vi "motors_id.vi"() -> ()   [LabVIEW 2019]
uses:
  Control 1.ctl
  <vilib>/Analysis/Matrix/Datatypes/RealMatrix.ctl
  <vilib>/userDefined/High Color/IMAQdx.ctl
  <vilib>/Platform/TimedLoop/XDataNode/timing_clust.ctl
  <vilib>/Platform/TimedLoop/XDataNode/nitl_modes.ctl
  <vilib>/Platform/TimedLoop/XDataNode/wakeup.ctl
  <vilib>/myRIO/Instrument Drivers/Onboard IO/AO/typedefs/AO Reference.ctl
  <vilib>/myRIO/Common/Instrument Driver Framework/Utilities/typedefs/myRIO Generic Hardware Reference.ctl
  <vilib>/myRIO/Common/Instrument Driver Framework/Utilities/typedefs/Hardware Version Enum.ctl
  <vilib>/myRIO/Common/Instrument Driver Framework/Utilities/typedefs/myRIO v1.0 Reference.ctl
  <vilib>/myRIO/Common/Instrument Driver Framework/Utilities/typedefs/Generic FPGA Reference.ctl
  <vilib>/myRIO/Common/Instrument Driver Framework/myRIO v1.0/AO/typedefs/AO Channels List.ctl
  <vilib>/myRIO/Common/Instrument Driver Framework/myRIO v1.0/AO/typedefs/AO Channels Enum.ctl
  <vilib>/myRIO/Common/Instrument Driver Framework/Utilities/typedefs/Analog Scaling Constants List.ctl
  <vilib>/myRIO/Common/Instrument Driver Framework/Utilities/typedefs/Analog Scaling Constants.ctl
  <vilib>/userDefined/High Color/nirio_resource_hc.ctl
  <vilib>/myRIO/Common/Instrument Driver Framework/myRIO v1.0/Encoder/typedefs/Encoder Signal Mode.ctl
  <vilib>/myRIO/Instrument Drivers/Onboard IO/Encoder/typedefs/Encoder Reference.ctl
  <vilib>/myRIO/Common/Instrument Driver Framework/myRIO v1.0/Encoder/typedefs/Encoder Channels Enum.ctl
  <vilib>/myRIO/Common/Instrument Driver Framework/myRIO v1.0/Encoder/typedefs/Encoder Configuration v1.0.ctl
  <vilib>/myRIO/Common/Instrument Driver Framework/Utilities/vis/Is FPGA Ref Available.vi
  <vilib>/myRIO/Common/Instrument Driver Framework/myRIO v1.0/AO/vis/myRIO v1.1 Open AO.vi
  <vilib>/myRIO/Instrument Drivers/Onboard IO/AO/vis/Write.vi
  <vilib>/myRIO/Common/Instrument Driver Framework/myRIO v1.0/Encoder/vis/myRIO v1.1 Open Encoder.vi
  <vilib>/myRIO/Instrument Drivers/Onboard IO/Encoder/vis/Read.vi
  <vilib>/myRIO/Common/Instrument Driver Framework/Utilities/vis/Validate Channels.vi
  <vilib>/myRIO/Common/Instrument Driver Framework/myRIO v1.0/AO/vis/myRIO v1.0 Reserve AO.vi
  <vilib>/myRIO/Common/Instrument Driver Framework/myRIO v1.0/Encoder/vis/myRIO v1.0 Reserve Encoder.vi
  <vilib>/myRIO/Common/Instrument Driver Framework/myRIO v1.0/AO/vis/myRIO v1.0 Build MUX Configuration AO.vi
  <vilib>/myRIO/Common/Instrument Driver Framework/myRIO v1.0/Resource Manager/vis/myRIO v1.0 Reserve Channel List.vi
  <vilib>/myRIO/Common/Instrument Driver Framework/myRIO v1.0/Encoder/vis/myRIO v1.0 Build MUX Configuration Encoder.vi
  <vilib>/myRIO/Common/Instrument Driver Framework/myRIO v1.0/Resource Manager/vis/myRIO v1.0 Reserve Channel.vi
  <vilib>/myRIO/Common/Instrument Driver Framework/myRIO v1.0/Resource Manager/vis/myRIO v1.0 Unreserve Channel.vi
  <vilib>/myRIO/Common/Instrument Driver Framework/myRIO v1.0/Resource Manager/vis/myRIO v1.0 Create Configuration List.vi
  <vilib>/myRIO/Common/Instrument Driver Framework/myRIO v1.0/Resource Manager/vis/myRIO v1.0 Build Mutex Name.vi
  <vilib>/Utility/VariantDataType/GetNumericInfo.vi
  <vilib>/Utility/error.llb/Error Cluster From Error Code.vi
  <vilib>/myRIO/Common/Instrument Driver Framework/myRIO v1.0/myRIO v1.1 Open.vi
  <vilib>/myRIO/Common/Instrument Driver Framework/myRIO v1.0/AO/vis/myRIO v1.0 Get Scaling Constants AO.vi
  <vilib>/myRIO/Common/Instrument Driver Framework/Utilities/vis/IO Manager.vi
  <vilib>/myRIO/Common/Instrument Driver Framework/Utilities/vis/Configuration Manager.vi
  <vilib>/myRIO/Common/Instrument Driver Framework/myRIO v1.0/myRIO v1.0 Close.vi
  <vilib>/myRIO/Common/Instrument Driver Framework/myRIO v1.0/AO/vis/myRIO v1.0 Write AO.vi
  <vilib>/Utility/file.llb/Write Delimited Spreadsheet (DBL).vi
  <vilib>/myRIO/Common/Instrument Driver Framework/myRIO v1.0/Resource Manager/vis/myRIO v1.0 Configure IO.vi
  <vilib>/myRIO/Common/Instrument Driver Framework/myRIO v1.0/Encoder/vis/myRIO v1.0 Configure Encoder.vi
  <vilib>/myRIO/Common/Instrument Driver Framework/myRIO v1.0/Encoder/vis/myRIO v1.0 Read Encoder.vi
  <vilib>/platform/TimedLoop/XDataNode/XDataNode.xnode
  <vilib>/myRIO/Express VI/Onboard IO/AO/AO Express VI.xnode
  <vilib>/myRIO/Instrument Drivers/Onboard IO/AO/vis/myRIO AO Open.xnode
  <vilib>/myRIO/Express VI/Onboard IO/Encoder/Encoder Express VI.xnode
  <vilib>/myRIO/Instrument Drivers/Onboard IO/Encoder/vis/myRIO Encoder Open.xnode
  <vilib>/myRIO/Common/Instrument Driver Framework/myRIO v1.0/Encoder/typedefs/Encoder Count Direction Enum.ctl
  <vilib>/Platform/TimedLoop/XDataNode/XDNodeRunTimeDep.lvlib
  <vilib>/myRIO/Instrument Drivers/Onboard IO/AO/AO.lvlib
  <vilib>/vision/driver/NI_Vision_Acquisition_Software.lvlib
  <vilib>/myRIO/Instrument Drivers/Onboard IO/Encoder/Encoder.lvlib
  <vilib>/vision/NI_Vision_Development_Module.lvlib
  <vilib>/Analysis/Matrix/NI_Matrix.lvlib
panel:
  in  "x_a":dbl(slide) step=1.0 scale=-45.0..45.0
  in  "y_a":dbl(slide) step=1.0 scale=-45.0..45.0
  in  "record_name":string
  out "record":T1
  out "step_recorded":dbl
  in  "stop_recording":bool
  in  "start_recording":bool
  out "recording":bool
  out "record_t":dbl[](array[numeric])
  out "target_angle_y_a_target":dbl(knob) scale=-45.0..45.0
  out "target_angle_x_a_target":dbl(knob) scale=-45.0..45.0
  in  "p_ki":dbl=-1.0
  in  "p_kd":dbl=-2000.0
  in  "p_kp":dbl
  out "y_angle":dbl(knob) scale=-45.0..45.0
  out "x_angle":dbl(knob) scale=-45.0..45.0
  out "y_error":dbl
  out "x_error":dbl
  in  "y_target":dbl(slide) scale=-1.0..1.0
  in  "x_target":dbl(slide) scale=-1.0..1.0
  out "y":dbl
  out "x":dbl
  out "camera":T2(plugin-control)
  in  "threshold":cluster{"Lower value":sgl, "Upper value":sgl}={"Lower value"=189.0, "Upper value"=255.0} {"Upper value" format="%.2f"; "Lower value" format="%.2f"}
  out "threshold":T2(plugin-control)
  out "x-y":u32
  out "y_input":dbl
  in  "a_ki":dbl=0.0003
  out "y_angle_error":dbl
  in  "a_kd":T3=-2.0
  in  "a_kp":dbl=0.12
  out "x_angle_error":dbl
  in  "stop":bool
  out "x_input":dbl
  in  "reset":bool
  in  "dt":dbl=70.0
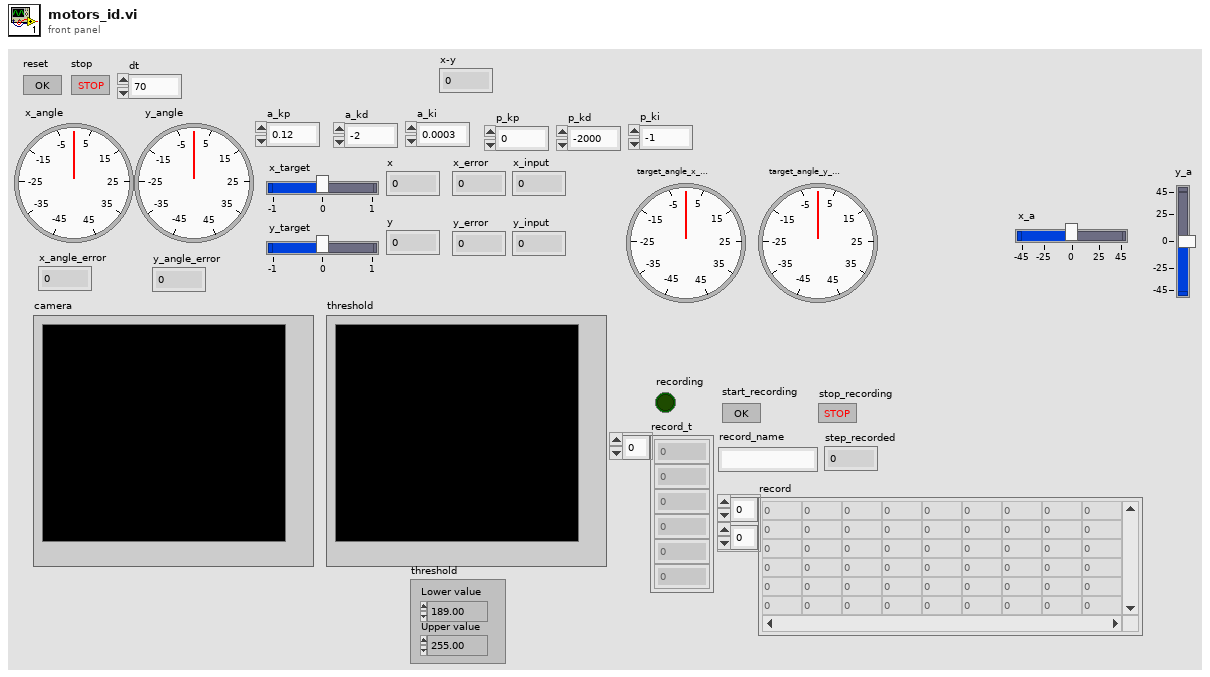
[diagram p1: front panel]
types:
  T1 = typedef "NI_Matrix.lvlib/RealMatrix.ctl" = dbl[][]
  T2 = typedef "IMAQ Image.ctl" = refnum<image>
  T3 = typedef "Control 1.ctl" = dbl
  T4 = typedef "IMAQdx.ctl" = refnum<k21>
  T5 = typedef "XDNodeRunTimeDep.lvlib/timing_clust.ctl" = cluster{"Expected End [f-1]":u64, "Actual End [f-1]":u64, "Finished Late? [f-1]":bool, "Expected End [i-1]":u64, "Actual End [i-1]":u64, "Finished Late? [i-1]":bool, "Expected Start [i]":u64, "Actual Start [i]":u64, "Expected Start [f]":u64, "Actual Start [f]":u64, "Source Name":string, "Structure Name":string, "Period":i64, "Deadline":i64, "Offset":i64, "Start":i64, "Priority":i32, "Timeout":i32, "Mode":T6, "Wakeup Reason":T7, "Error":errorcluster, "Source Type":string, "Secondary Source Type":string, "Global End Time":u64, "Global Start Time":u64, "Frame Duration":u64, "Iteration Duration":u64, "Assigned CPU":i32, "I/O Scan Engine Mode":u32}
  T6 = typedef "XDNodeRunTimeDep.lvlib/nitl_modes.ctl" = enum32{"No Change", "Process missed periods, maintain original phase", "Discard missed periods, maintain original phase", "Process missed periods, ignore original phase", "Discard missed periods, ignore original phase"}
  T7 = typedef "XDNodeRunTimeDep.lvlib/wakeup.ctl" = enum32{"Normal", "Aborted", "Asynchronous wakeup", "Timing source error", "Timed loop error", "Timeout"}
  T8 = typedef "Encoder.lvlib/Encoder Reference.ctl" = cluster{"myRIO Reference":T9, "Encoder Channels Enum":T13}
  T9 = typedef "myRIO Generic Hardware Reference.ctl" = cluster{"myRIO Model":T10, "myRIO Hardware Reference":T11}
  T10 = typedef "Hardware Version Enum.ctl" = enum16{"Unknown", "myRIO-1900", "myRIO-1950", "roboRIO", "NI ELVIS RIO CM", "ELVIS III"}
  T11 = typedef "myRIO v1.0 Reference.ctl" = cluster{"Generic FPGA Reference":T12, "Allow multiple opens":bool}
  T12 = typedef "Generic FPGA Reference.ctl" = refnum<k20>
  T13 = typedef "Encoder Channels Enum.ctl" = enum16{"Not Connected", "C/ENC0", "C/ENC1", "A/ENC", "A/ENC0", "A/ENC1", "A/ENC2", "A/ENC3", "A/ENC4", "A/ENC5", "A/ENC6", "A/ENC7", "A/ENC8", "A/ENC9", "B/ENC", "B/ENC0", "B/ENC1", "B/ENC2", "B/ENC3", "B/ENC4", "B/ENC5", "B/ENC6", "B/ENC7", "B/ENC8", "B/ENC9", "DIO/ENC0", "DIO/ENC1", "DIO/ENC2", "DIO/ENC3", "DIO/ENC4"}
  T14 = typedef "Encoder Signal Mode.ctl" = enum16{"Quadrature phase signal", "Step and direction signal"}
  T15 = typedef "nirio_resource_hc.ctl" = tag
  T16 = typedef "AO.lvlib/AO Reference.ctl" = cluster{"myRIO Reference":T9, "AO Channel List":T17, "AO Scaling Constant List":T19}
  T17 = typedef "AO Channels List.ctl" = T18[]
  T18 = typedef "AO Channels Enum.ctl" = enum16{"Not Connected", "AudioOut/Left", "AudioOut/Right", "C/AO0", "C/AO1", "A/AO0", "A/AO1", "B/AO0", "B/AO1"}
  T19 = typedef "Analog Scaling Constants List.ctl" = T20[]
  T20 = typedef "Analog Scaling Constants.ctl" = cluster{"LSB Weight (Volts)":dbl, "Offset (Volts)":dbl, "Signed?":bool}
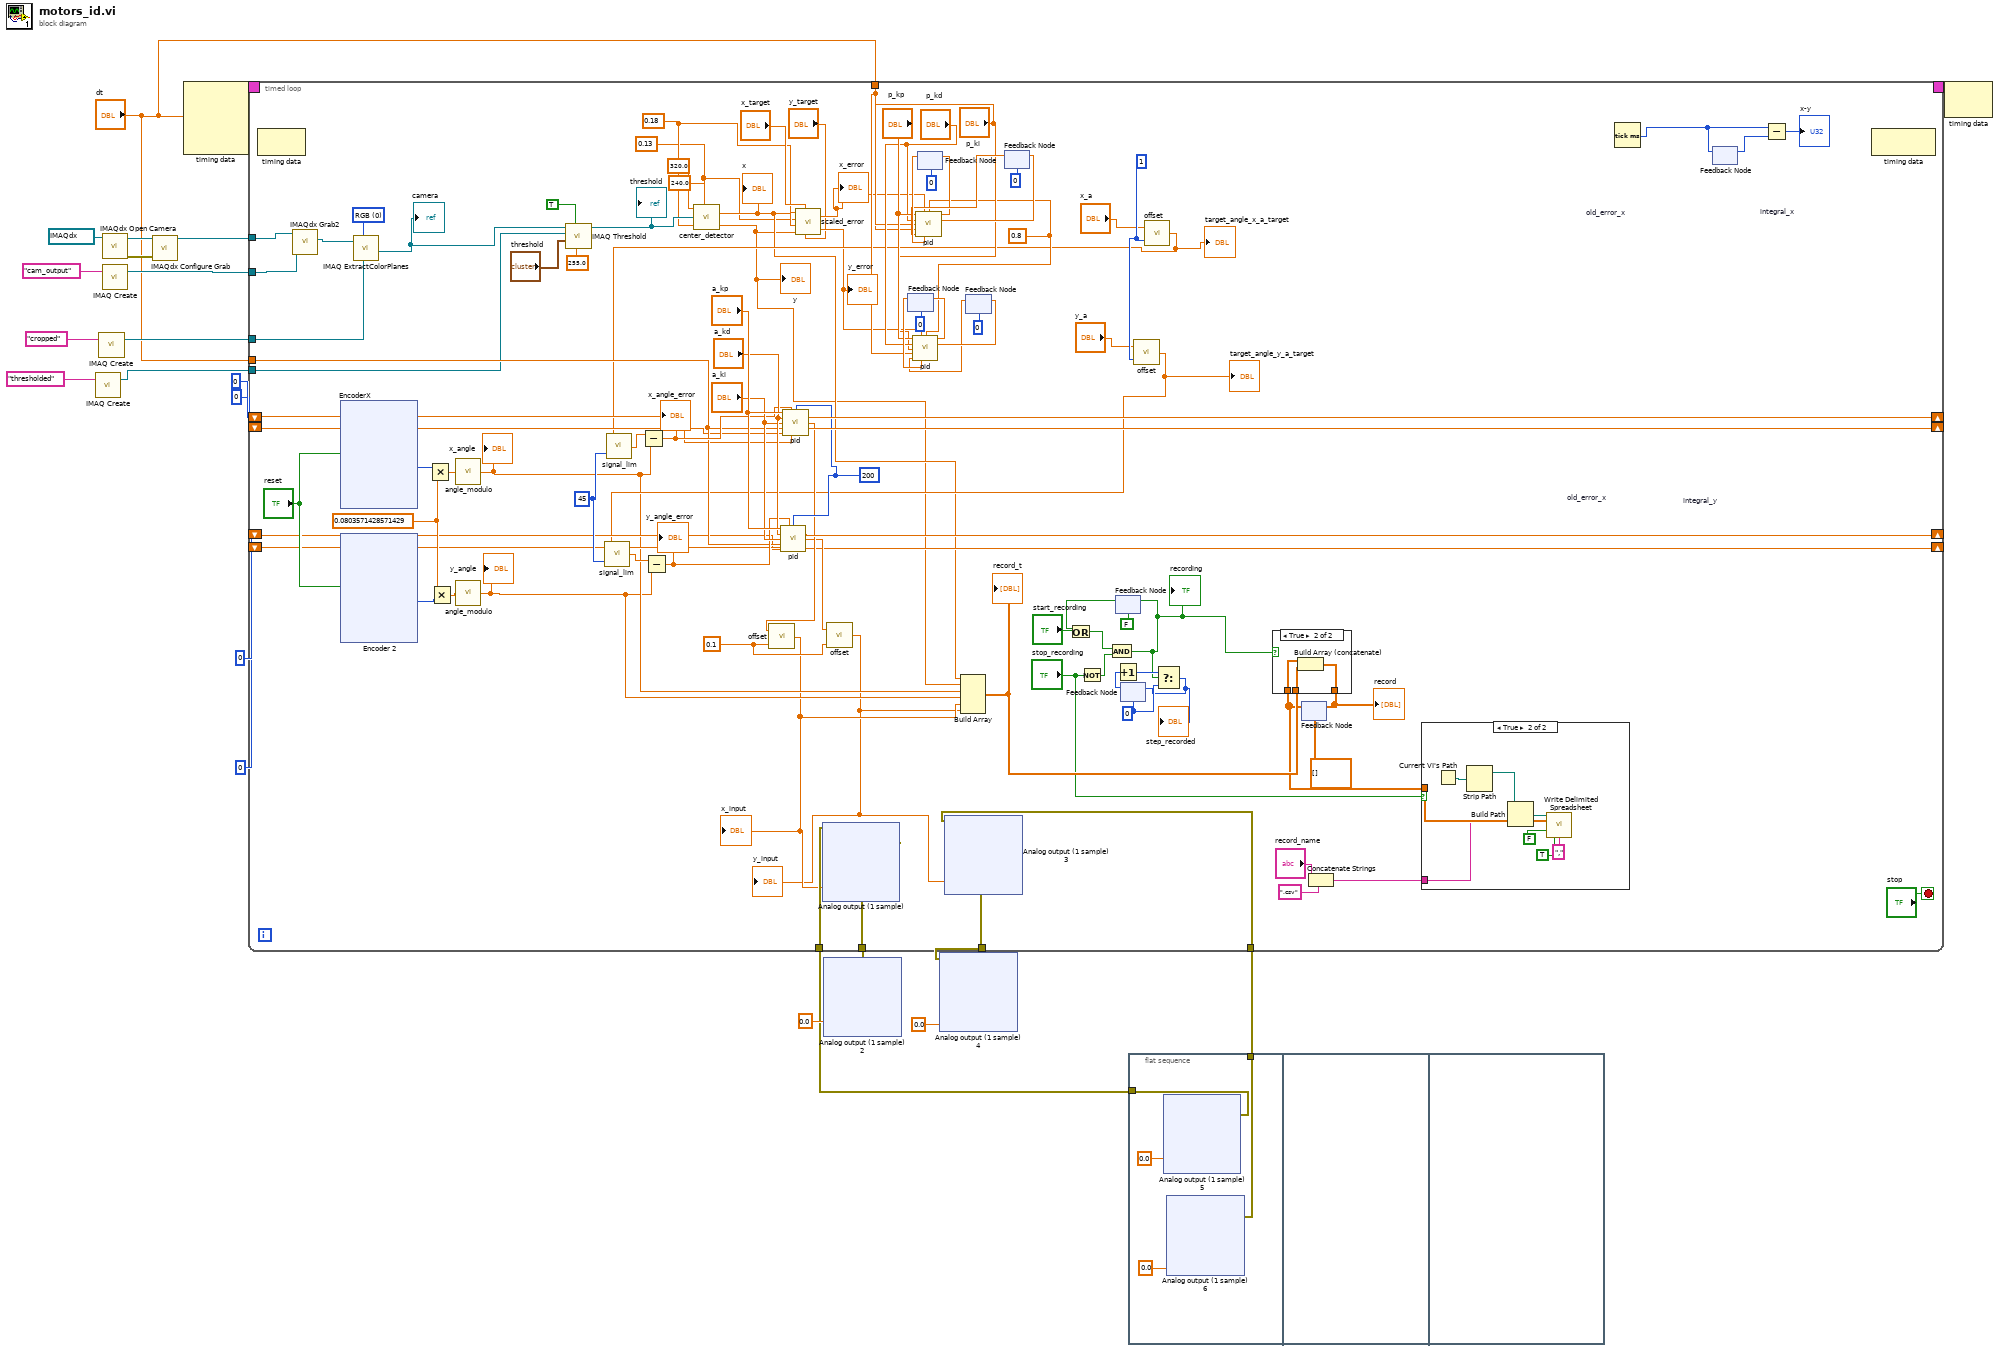
[diagram p0: block diagram]
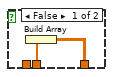
[diagram p3: hidden frame]
diagram:
  n1 = call "IMAQ Create"("Image Name"="thresholded") -> ("New Image"=w2:T2)  [unwired: 4 in, 1 out]
  n2 = call "IMAQ Create"("Image Name"="cropped") -> ("New Image"=w4:T2)  [unwired: 4 in, 1 out]
  n3 = call <vilib>:"IMAQdx Open Camera.vi"("Session In"=T4 "cam2") -> ("error out"=w15:errorcluster, "Session Out"=w16:T4)  [unwired: 9 in]
  n4 = call "IMAQ Create"("Image Name"="cam_output") -> ("New Image"=w17:T2)  [unwired: 4 in, 1 out]
  n5 = call <vilib>:"IMAQdx Configure Grab.vi"("error in"=w15, "Session In"=w16) -> ("Session Out"=w18:T4)  [unwired: 8 in, 1 out]
  n6 = node-c288("dt") -> (w23:T5)  [unwired: 3 in]
  n7 = timed-loop {
    timing: w23 -> [_]
    timing-out: [_] -> w22
    tunnel: w18 -> [w123]
    tunnel: w17 -> [w122]
    shift-right: [w100] -> _
    shift-left: 0 -> [w105]
    shift-right: [w99] -> _
    shift-left: 0 -> [w104]
    shift-right: [w65] -> _
    shift-left: 0 -> [w103]
    shift-right: [w101] -> _
    shift-left: 0 -> [w102]
    tunnel: "dt" -> [w106]
    tunnel: [w98] -> w9
    tunnel: [w94] -> w8
    tunnel: w7 -> [w93]
    tunnel: w6 -> [w92]
    tunnel: w4 -> [w37]
    tunnel: w2 -> [w41]
    tunnel: "dt" -> [w73]
    stop <- "stop" stop-if-true
    w26 = 0.13 ("m_y")
    w27 = 0.18 ("m_x")
    w40 = u16 0 items=["RGB", "HSL", "HSV", "HSI"] ("Color Mode")
    w52 = 0
    w66 = 1
    w70 = 0.1
    w71 = 200
    w72 = 0.8
    w112 = 45
    w120 = 0.0803571428571429
    n8 = node-c288() -> ()  [unwired: 1 in, 1 out]
    n9 = call <vilib>:"IMAQdx Grab2.vi"("Image In"=w122, "Session In"=w123) -> ("Image Out"=w39:T2)  [unwired: 6 in, 3 out]
    n10 = xnode "EncoderX"("Reset Counter"="reset") -> ("Counter Value"=w121:i32)  [unwired: 1 in, 3 out]
    n11 = xnode "Encoder 2"("Reset Counter"="reset") -> ("Counter Value"=w119:i32)  [unwired: 1 in, 3 out]
    n12 = call "IMAQ ExtractColorPlanes"("Blue or Luma or Val or Inten Plane"=w37, "Color Mode"=w40, "Image Src"=w39) -> ("Blue or Luma or Val or Inten Plane out"=w38:T2)  [unwired: 5 in, 3 out]
    "camera" <- w38
    n13 = Multiply(x=w121, y=w120) -> (x*y=w116:dbl)
    n14 = Multiply(x=w120, y=w119) -> (x*y=w115:dbl)
    n15 = call "angle_modulo.vi"("alpha"=w116) -> ("alpha_prime"=w63:dbl)
    "x_angle" <- w63
    n16 = call "angle_modulo.vi"("alpha"=w115) -> ("alpha_prime"=w62:dbl)
    "y_angle" <- w62
    n17 = call "IMAQ Threshold"("Replace Value"=sgl 255.0, "Keep/Replace Value (Replace)"=TRUE, "Range"="threshold", "Image Dst"=w41, "Image Src"=w38) -> ("Image Dst Out"=w34:T2)  [unwired: 5 in, 1 out]
    "threshold" <- w34
    n18 = call "center_detector.vi"("px_x"=320.0, "px_y"=240.0, "Image"=w34, "m_x"=w27, "m_y"=w26) -> ("x"=w29:dbl, "y"=w28:dbl)
    "x" <- w29
    "y" <- w28
    n19 = call "scaled_error.vi"("y_target"="y_target", "x_target"="x_target", "y"=w28, "x"=w29, "m_y"=w26, "m_x"=w27) -> ("err_y"=w33:dbl, "err_x"=w32:dbl)
    "x_error" <- w32
    "y_error" <- w33
    n20 = feedback #1 "old_error_x"(0) -> (w79:dbl)
    n21 = feedback #2 "old_error_x"(0) -> (w84:dbl)
    n22 = feedback #3 "integral_y"(0) -> (w77:dbl)
    n23 = call "pid.vi"("kp"="p_kp", "err"=w33, "lim"=w72, "kd"="p_kd", "ki"="p_ki", "dt"=w73, "intergral"=w77, "old_err"=w79) -> ("curr_err"=w80:dbl, "curr_integral"=w78:dbl)  [unwired: 5 in, 1 out]
    n24 = feedback-in #1(w80) -> ()
    n25 = feedback-in #3(w78) -> ()
    n26 = feedback #4 "integral_x"(0) -> (w82:dbl)
    n27 = call "pid.vi"("kp"="p_kp", "err"=w32, "lim"=w72, "kd"="p_kd", "ki"="p_ki", "dt"=w73, "intergral"=w82, "old_err"=w84) -> ("curr_err"=w81:dbl, "curr_integral"=w83:dbl)  [unwired: 5 in, 1 out]
    n28 = feedback-in #2(w81) -> ()
    n29 = feedback-in #4(w83) -> ()
    n30 = Not(x="stop_recording") -> (.not. x?=w56:bool)
    n31 = feedback #5(FALSE) -> (w58:bool)
    n32 = Or(x=w58, y="start_recording") -> (x .or. y?=w57:bool)
    n33 = And(x=w57, y=w56) -> (x .and. y?=w50:bool)
    "recording" <- w50
    n34 = feedback-in #5(w50) -> ()
    n35 = feedback #6(w52) -> (w54:i32)
    n36 = Increment(x=w54) -> (x+1=w53:i32)
    n37 = call "offset.vi"("offset"=w66, "x"="y_a") -> ("y"=w67:dbl)
    "target_angle_y_a_target" <- w67
    n38 = call "signal_lim.vi"("lim"=w112, "x"=w67) -> ("y"=w113:dbl)
    n39 = Subtract(x=w113, y=w62) -> (x-y=w107:dbl)
    "y_angle_error" <- w107
    n40 = call "pid.vi"("kp"="a_kp", "err"=w107, "lim"=w71, "kd"="a_kd", "ki"="a_ki", "dt"=w106, "intergral"=w102, "old_err"=w103) -> ("curr_err"=w65:dbl, "curr_integral"=w101:dbl, "y"=w68:dbl)  [unwired: 5 in]
    n41 = call "offset.vi"("offset"=w70, "x"=w68) -> ("y"=w60:dbl)
    "y_input" <- w60
    n42 = xnode "Analog output (1 sample) 3"("C/AO1 (AO1)"=w60, "error in (no error)"=w92) -> ("error out"=w94:errorcluster)
    n43 = call "offset.vi"("offset"=w66, "x"="x_a") -> ("y"=w64:dbl)
    "target_angle_x_a_target" <- w64
    n44 = call "signal_lim.vi"("lim"=w112, "x"=w64) -> ("y"=w114:dbl)
    n45 = Subtract(x=w114, y=w63) -> (x-y=w108:dbl)
    "x_angle_error" <- w108
    n46 = call "pid.vi"("kp"="a_kp", "err"=w108, "lim"=w71, "kd"="a_kd", "ki"="a_ki", "dt"=w106, "intergral"=w104, "old_err"=w105) -> ("curr_err"=w100:dbl, "curr_integral"=w99:dbl, "y"=w69:dbl)  [unwired: 5 in]
    n47 = call "offset.vi"("offset"=w70, "x"=w69) -> ("y"=w61:dbl)
    "x_input" <- w61
    n48 = xnode "Analog output (1 sample)"("C/AO0 (AO0)"=w61, "error in (no error)"=w93) -> ("error out"=w98:errorcluster)
    n49 = Build Array(w29, w28, w63, w62, w61, w60) -> (w49:dbl[])
    "record_t" <- w49
    n50 = Select(t=w53, s=w50, f=w52) -> (s? t:f=w51:i32)
    "step_recorded" <- w51
    n51 = feedback-in #6(w51) -> ()
    n52 = feedback #7(T1 [] ("Real Matrix")) -> (w45:T1)
    n53 = case shown="True" w50 {
      tunnel: w45 -> [_ w136]
      tunnel: [w132 w135] -> w47
      tunnel: w49 -> [w133 w134]
      frame False {
        n54 = Build Array(w133) -> (w132:T1)
      }
      frame True {
        n55 = Build Array (concatenate)(w136, w134) -> (w135:T1)
      }
    }
    "record" <- w47
    n56 = feedback-in #7(w47) -> ()
    n57 = Concatenate Strings("record_name", ".csv") -> (w42:string)
    n58 = case shown="True" "stop_recording" {
      tunnel: w45 -> [_ w131]
      tunnel: w42 -> [_ w129]
      frame False {
      }
      frame True {
        n59 = Current VI's Path() -> (path=w127:path)
        n60 = Strip Path(path=w127) -> (stripped path=w126:path)  [unwired: 1 out]
        n61 = Build Path(base path=w126, name or relative path=w129) -> (appended path=w128:path)
        n62 = call-poly <vilib>:"Write Delimited Spreadsheet.vi"("file path (dialog if empty)"=w128, "2D data"=w131, "append to file? (new file:F)"=FALSE, "transpose? (no:F)"=TRUE, "delimiter (\\t)"="," ("delimiter (\\t)")) -> ()  [unwired: 9 in, 2 out]
      }
    }
    n63 = Tick Count (ms)() -> (millisecond timer value=w97:u32)
    n64 = feedback-in #8(w97) -> ()
    n65 = feedback #8() -> (w96:u32)  [unwired: 1 in]
    n66 = Subtract(x=w97, y=w96) -> (x-y=→"x-y":u32)
    n67 = node-c288() -> ()  [unwired: 1 in, 1 out]
  }
  n68 = xnode "Analog output (1 sample) 2"("C/AO0 (AO0)"=0.0, "error in (no error)"=w9) -> ()  [unwired: 1 out]
  n69 = xnode "Analog output (1 sample) 4"("C/AO1 (AO1)"=0.0, "error in (no error)"=w8) -> ()  [unwired: 1 out]
  n70 = flat-sequence {
    tunnel: [w306] -> w7
    tunnel: [w305] -> w6
    frame #0 {
      n71 = xnode "Analog output (1 sample) 5"("C/AO0 (AO0)"=0.0) -> ("error out"=w306:errorcluster)  [unwired: 1 in]
      n72 = xnode "Analog output (1 sample) 6"("C/AO1 (AO1)"=0.0) -> ("error out"=w305:errorcluster)  [unwired: 1 in]
    }
    frame #1 {
    }
    frame #2 {
    }
  }
  n73 = node-c288(w22) -> ()  [unwired: 1 out]
